vi "Test Invalid Registration - Server Error.vi"() -> (2 "Success":bool)   [LabVIEW 2024]
uses:
  Mock Sift Proxy Server/Mock Sift Proxy Server.lvclass
  Sift API/Sift Client.lvclass
  Sift API/Types/Data Type.ctl
  Sift Client.lvlib
panel:
  out "Server Error":errorcluster
  out "Error":errorcluster
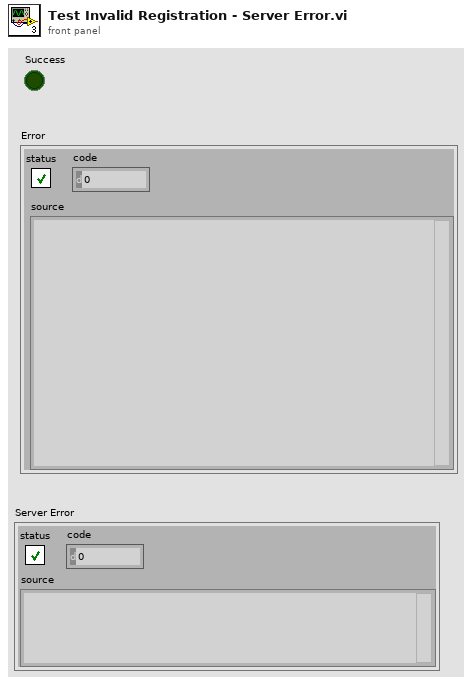
[diagram p1: front panel]
types:
  T1 = typedef "Sift Client.lvlib/Data Type.ctl" = enum8{"double", "float", "uint64", "int64", "uint32", "int32", "bool", "bit field", "enum"}
  T2 = typedef "Sift Client.lvlib/JSON Response.ctl" = cluster{"status":bool, "data":variant}
  T3 = typedef "Sift Client.lvlib/Channel Config.ctl" = cluster{"name":string, "data_type":T1, "description":string, "component":string, "unit":string, "bit_field_elements":T4[], "enum_types":T5[]}
  T4 = typedef "Sift Client.lvlib/Bit Field.ctl" = cluster{"index":u32, "bit_count":u32, "name":string}
  T5 = typedef "Sift Client.lvlib/Enum.ctl" = cluster{"Key":u32, "Name":string}
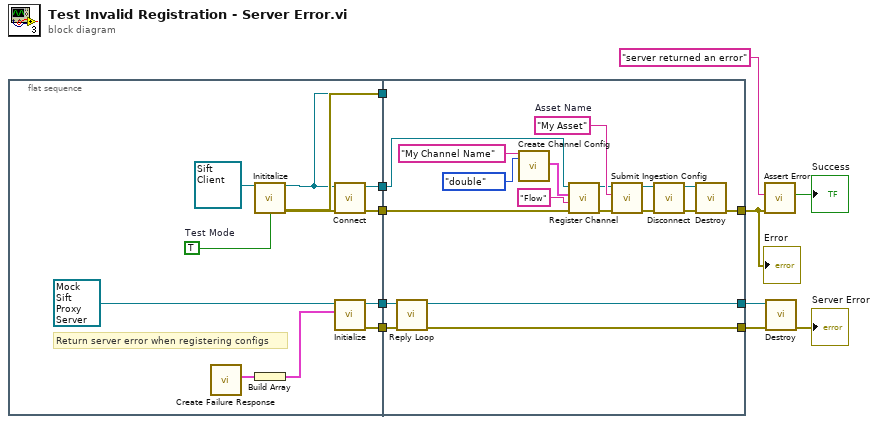
[diagram p0: block diagram]
diagram:
  n1 = flat-sequence {
    tunnel: [w22] -> w10
    tunnel: [w19] -> w8
    tunnel: [w18] -> w7
    tunnel: [w17] -> w6
    tunnel: [w16] -> w5
    tunnel: [w15] -> w4
    tunnel: [w30] -> w11
    tunnel: w10 -> [w31]
    tunnel: [w39] -> w9
    tunnel: w8 -> [_]
    tunnel: w7 -> [_]
    tunnel: w6 -> [w29]
    tunnel: w5 -> [w28]
    tunnel: w4 -> [w25]
    tunnel: [w24] -> w3
    frame #0 {
      w20 = TRUE  # Test Mode
      # "Return server error when registering configs"
      n2 = call "Create Failure Response.vi"() -> ("output cluster"=w13:T2)  [unwired: 11 in]
      n3 = call-dynamic "Inititalize.vi"("Sift Client in"=refnum<class "Sift Client.lvclass"> refnum ("Sift Client.lvlib:Sift Client.lvclass"), "Test Mode"=w20) -> ("Sift Client out"=w18:refnum<class "Sift Client.lvclass">, "error out"=w19:errorcluster)  [unwired: 12 in]
      n4 = Build Array(w13) -> (w14:T2[])
      n5 = call-dynamic "Connect.vi"("error in (no error)"=w19, "Sift Client in"=w18) -> ("error out"=w17:errorcluster, "Sift Client out"=w16:refnum<class "Sift Client.lvclass">)  [unwired: 7 in, 1 out]
      n6 = call-dynamic "Initialize.vi"("Mock Replies"=w14, "Mock Sift Proxy Server in"=refnum<class "Mock Sift Proxy Server.lvclass"> refnum ("Mock Sift Proxy Server.lvclass")) -> ("error out"=w15:errorcluster, "Mock Sift Proxy Server out"=w22:refnum<class "Mock Sift Proxy Server.lvclass">)  [unwired: 8 in]
    }
    frame #1 {
      w35 = "My Asset"  # Asset Name
      n7 = call-dynamic "Reply Loop.vi"("error in (no error)"=w25, "Mock Sift Proxy Server in"=w31) -> ("error out"=w24:errorcluster, "Mock Sift Proxy Server out"=w30:refnum<class "Mock Sift Proxy Server.lvclass">)  [unwired: 8 in]
      n8 = call "Create Channel Config.vi"("Name"="My Channel Name", "Data Type"=Data_Type."double" ("Enum")) -> ("Output"=w36:T3)  [unwired: 17 in]
      n9 = call-dynamic "Register Channel.vi"("error in (no error)"=w29, "Flow Name"="Flow", "Channel Config"=w36, "Sift Client in"=w28) -> ("error out"=w40:errorcluster, "Sift Client out"=w33:refnum<class "Sift Client.lvclass">)  [unwired: 6 in]
      n10 = call-dynamic "Submit Ingestion Config.vi"("error in (no error)"=w40, "Asset Name"=w35, "Sift Client in"=w33) -> ("error out"=w41:errorcluster, "Sift Client out"=w32:refnum<class "Sift Client.lvclass">)  [unwired: 6 in, 1 out]
      n11 = call-dynamic "Disconnect.vi"("error in (no error)"=w41, "Sift Client in"=w32) -> ("error out"=w26:errorcluster, "Sift Client out"=w27:refnum<class "Sift Client.lvclass">)  [unwired: 8 in]
      n12 = call-dynamic "Destroy.vi"("error in (no error)"=w26, "Sift Client in"=w27) -> ("error out"=w39:errorcluster)  [unwired: 8 in, 1 out]
    }
  }
  n13 = call "Assert Error.vi"("Error"=w9, "Error String"="server returned an error") -> ("Success"=→"Success":bool)  [unwired: 9 in]
  n14 = call-dynamic "Destroy.vi"("error in (no error)"=w3, "Mock Sift Proxy Server in"=w11) -> ("error out"=→"Server Error":errorcluster)  [unwired: 8 in, 1 out]
  "Error" <- w9
